vi "Host Main.vi"() -> ()   [LabVIEW 2014]
doc: "This application launches and executes the Tag Bus Data framework configuration for the specified target alias. This is a simple example of the framework API functions, but may also be a suitable starting point for a Host UI or Thick Client that is running a local version of the framework."
uses:
  <vilib>/NI/Module Execution Interface/Engine Runtime/Execution States.ctl
  <vilib>/NI/Module Execution Interface/Engine Runtime/Fault.ctl
  <vilib>/NI/Tag Bus Module Framework/runtime/error classification.ctl
  <vilib>/NI/Current Value Table/DataTypes/Double_Read.vi
  <vilib>/NI/Current Value Table/DataTypes/Array of Double_Read.vi
  <vilib>/NI/Current Value Table/Type to Enum.vi
  <vilib>/NI/Current Value Table/DataTypes/Double_Type To Enum.vi
  <vilib>/NI/Current Value Table/DataTypes/Array of Double_Type To Enum.vi
  <vilib>/NI/Current Value Table/FGVs/CVT Globals.vi
  <vilib>/NI/Current Value Table/FGVs/Tag Memory.vi
  <vilib>/NI/Current Value Table/Memory Block.vi
  <vilib>/NI/Current Value Table/DataTypes/Double_Memory Block.vi
  <vilib>/NI/Current Value Table/DataTypes/Array of Double_Memory Block.vi
  <vilib>/userdefined/High Color/nirio_resource_hc.ctl
  <vilib>/NI/Module Execution Interface/Engine Runtime/Engine Runtime Interface.lvclass
  <vilib>/NI/DCAF/Tag Editor Core/Framework Configuration Classes/target runtime/PL_Target Runtime.lvclass
  <vilib>/NI/Tag Bus Module Framework/FPGA manager/FPGA manager.lvlib
  <vilib>/rvi/interface/nirviOpenFPGA/nirviOpenFPGA.xnode
  <vilib>/NI/Tag Bus Module Framework/FPGA manager/methods.ctl
  <vilib>/NI/Current Value Table/Current Value Table.lvlib
  <vilib>/NI/Tag Bus Module Framework/runtime/TBM module execution interface.lvclass
panel:
  out "DiskUsage":dbl
  out "DiskUsagePercentage":dbl
  out "CPU_Usage":dbl[](array[numeric])
  out "CPU_UsageTotal":dbl
  out "MemoryUsagePercentage":dbl
  out "MemoryUsage":dbl
  out "engine status":T4(array[cluster])
  in  "stop":bool
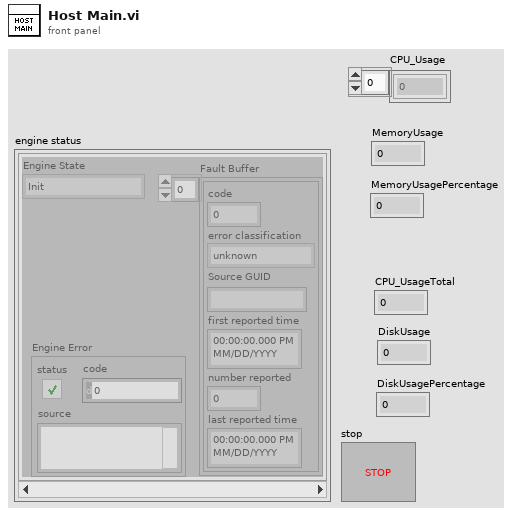
[diagram p1: front panel]
types:
  T1 = typedef "Engine Runtime Interface.lvclass/Execution States.ctl" = enum16{"Init", "Pre-Operational", "Safe-Operational", "Operational", "Stopped"}
  T2 = typedef "Engine Runtime Interface.lvclass/Fault.ctl" = cluster{"code":i32, "error classification":T3, "Source GUID":string, "first reported time":timestamp, "number reported":u32, "last reported time":timestamp}
  T3 = typedef "TBM module execution interface.lvclass/error classification.ctl" = enum16{"unknown", "none", "trivial", "recoverable", "critical"}
  T4 = cluster{"Engine State":T1, "Fault Buffer":T2[], "Engine Error":errorcluster}[]
  T5 = typedef "FPGA manager.lvlib/methods.ctl" = enum16{"initialize bitfile", "cache bitfile", "locate bitfile", "close bitfile", "clear manager"}
  T6 = typedef "nirio_resource_hc.ctl" = tag
  T7 = cluster{"Engine State":T1, "faults":T2[], "Engine Error":errorcluster}
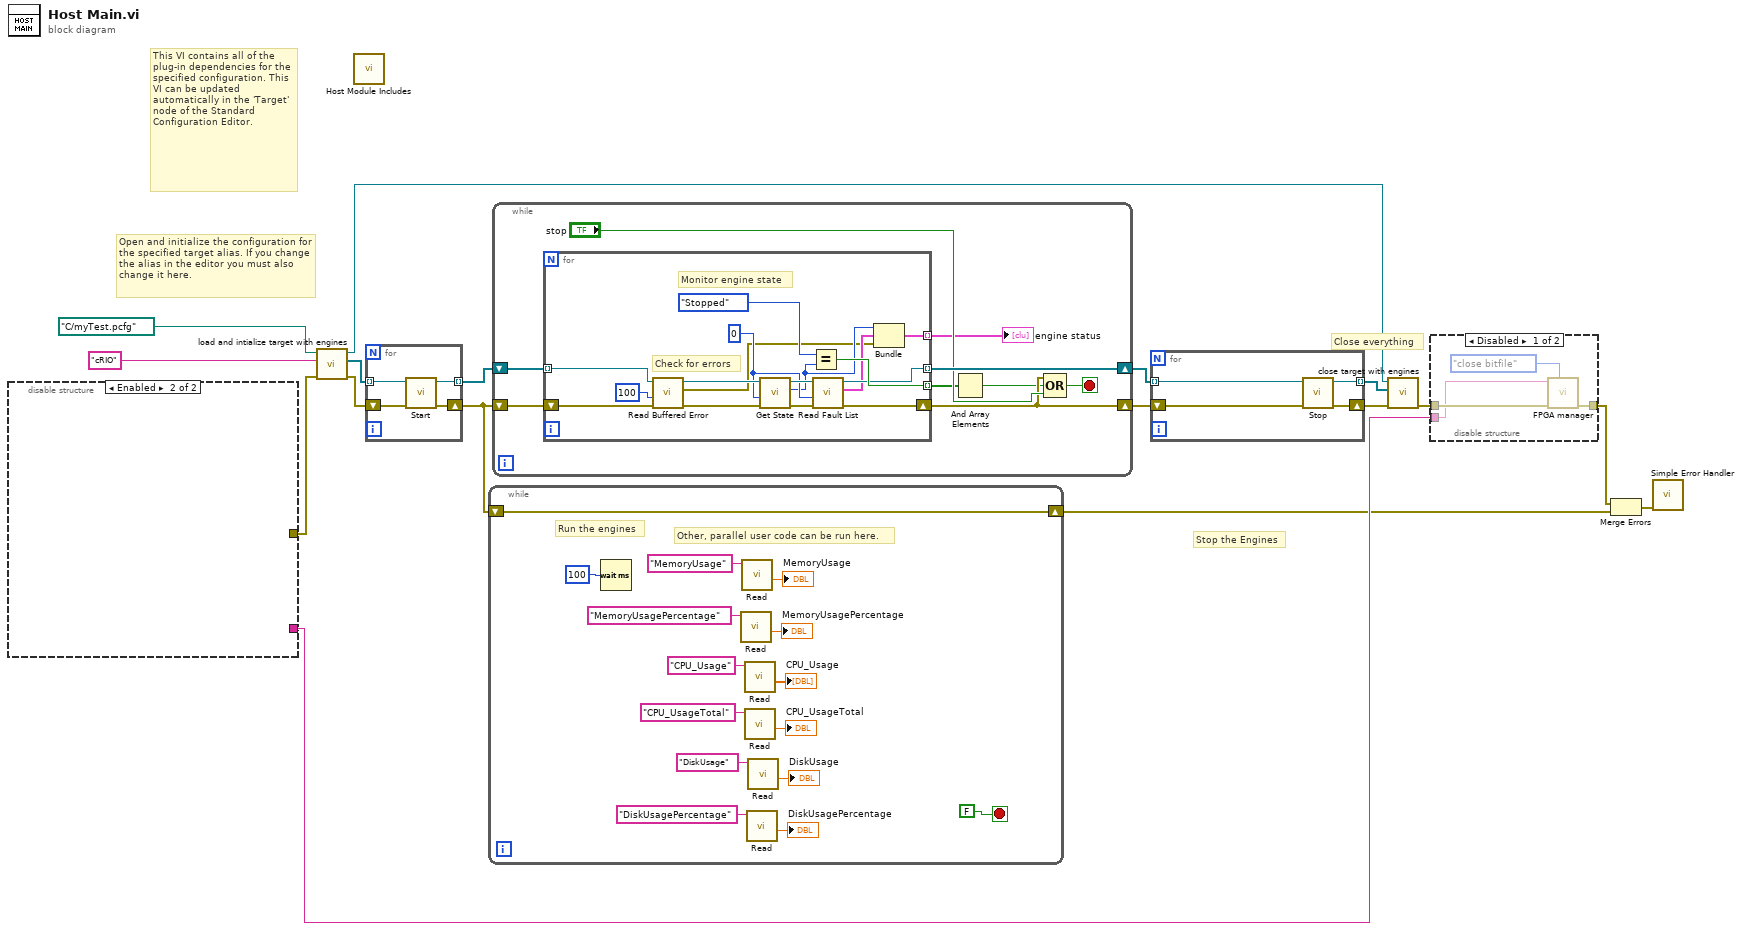
[diagram p0: block diagram]
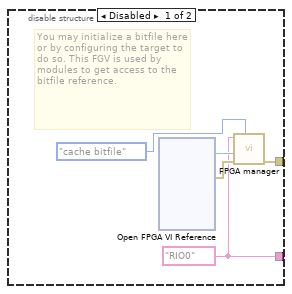
[diagram p3: hidden frame]
diagram:
  # "Open and initialize the configuration for the specified target alias. If you change the alias in the editor you must also change it here."
  # "Close everything"
  # "Stop the Engines"
  # "This VI contains all of the plug-in dependencies for the specified configuration. This VI can be updated automatically in the 'Target' node of the Standard Configuration Editor."
  # "Run the engines"
  n1 = disable-structure shown="Enabled" {
    disable-tunnel: [w22 _] -> w7
    disable-tunnel: [w18 _] -> w6
    frame Disabled {
      w18 = T6 "RIO0" ("RIO resource")
      # "You may initialize a bitfile here or by configuring the target to do so. This FGV is used by modules to get access to the bitfile reference."
      n2 = xnode "Open FPGA VI Reference"() -> ("FPGA VI Reference Out"=w20:refnum<k20>, "error out"=w21:errorcluster)  [unwired: 2 in]
      n3 = call <vilib>:"FPGA manager.vi"("action"=methods."cache bitfile", "error in"=w21, "bitfile to cache"=w20, "RIO resource"=w18) -> ("error out"=w22:errorcluster)  [unwired: 5 in, 2 out]
    }
    frame Enabled {
    }
  }
  n4 = call <vilib>:"load and intialize target with engines.vi"("error in"=w7, "target alias"="cRIO", "file path"=path "C:/myTest.pcfg" ("configuration file path")) -> ("error out"=w14:errorcluster, "engine runtime interfaces"=w13:refnum<class "Engine Runtime Interface.lvclass">[], "target runtime"=w10:refnum<class "PL_Target Runtime.lvclass">)  [unwired: 6 in]
  n5 = call "Host Module Includes.vi"() -> ()  [unwired: 12 in]
  n6 = for {
    tunnel: [w26] -> w17 mode=indexing
    tunnel: w13 -> [w23] mode=indexing
    shift-right: [w25] -> w5
    shift-left: w14 -> [w24]
    n7 = call-dynamic "Start.vi"("error in"=w24, "Engine Runtime Interface in"=w23) -> ("error out"=w25:errorcluster, "Engine Runtime Interface out"=w26:refnum<class "Engine Runtime Interface.lvclass">)  [unwired: 8 in]
  }
  n8 = while {
    shift-right: [w39] -> w4
    shift-left: w5 -> [w39]
    stop <- FALSE stop-if-true
    # "Other, parallel user code can be run here."
    n9 = Wait (ms)(milliseconds to wait=u32 100) -> ()  [unwired: 1 out]
    n10 = call-poly <vilib>:"Read.vi"("Tag Name"="MemoryUsagePercentage") -> ("Value"=→"MemoryUsagePercentage":dbl)  [unwired: 9 in, 1 out]
    n11 = call-poly <vilib>:"Read.vi"("Tag Name"="MemoryUsage") -> ("Value"=→"MemoryUsage":dbl)  [unwired: 9 in, 1 out]
    n12 = call-poly <vilib>:"Read.vi"("Tag Name"="CPU_Usage") -> ("Value"=→"CPU_Usage":dbl[])  [unwired: 9 in, 1 out]
    n13 = call-poly <vilib>:"Read.vi"("Tag Name"="CPU_UsageTotal") -> ("Value"=→"CPU_UsageTotal":dbl)  [unwired: 9 in, 1 out]
    n14 = call-poly <vilib>:"Read.vi"("Tag Name"="DiskUsagePercentage") -> ("Value"=→"DiskUsagePercentage":dbl)  [unwired: 9 in, 1 out]
    n15 = call-poly <vilib>:"Read.vi"("Tag Name"="DiskUsage") -> ("Value"=→"DiskUsage":dbl)  [unwired: 9 in, 1 out]
  }
  n16 = while {
    shift-right: [w48] -> w16
    shift-left: w17 -> [w50]
    shift-right: [w45] -> w15
    shift-left: w5 -> [w49]
    stop <- w46 stop-if-true
    n17 = for {
      tunnel: w50 -> [w66] mode=indexing
      tunnel: [w57] -> w48 mode=indexing
      tunnel: [w61] -> w43 mode=indexing
      shift-right: [w56] -> w45
      shift-left: w49 -> [w65]
      tunnel: [w51] -> w44 mode=indexing
      w55 = 0 ("timeout (-1)")
      # "Monitor engine state"
      # "Check for errors"
      n18 = call-dynamic "Read Buffered Error.vi"("error in"=w65, "timeout in ms (0)"=100, "Engine Runtime Interface in"=w66) -> ("error out"=w63:errorcluster, "Engine Error"=w52:errorcluster, "Engine Runtime Interface out"=w64:refnum<class "Engine Runtime Interface.lvclass">)  [unwired: 6 in]
      n19 = call-dynamic "Get State.vi"("error in"=w63, "timeout (-1)"=w55, "Engine Runtime Interface in"=w64) -> ("error out"=w59:errorcluster, "Engine State"=w54:T1, "Engine Runtime Interface out"=w58:refnum<class "Engine Runtime Interface.lvclass">)  [unwired: 6 in]
      n20 = Equal?(x=Execution_States."Stopped" ("Engine State"), y=w54) -> (x = y?=w61:bool)
      n21 = call-dynamic "Read Fault List.vi"("error in"=w59, "timeout (-1)"=w55, "Engine Runtime Interface in"=w58) -> ("error out"=w56:errorcluster, "faults"=w53:T2[], "Engine Runtime Interface out"=w57:refnum<class "Engine Runtime Interface.lvclass">)  [unwired: 6 in]
      n22 = Bundle("Engine State"=w54, "faults"=w53, "Engine Error"=w52) -> (w51:T7)  [unwired: 1 in]
    }
    "engine status" <- w44
    n23 = And Array Elements(Boolean array=w43) -> (logical AND=w42:bool)
    n24 = Compound Arithmetic op=OR(w45, w42, "stop") -> (w46:bool)
  }
  n25 = for {
    tunnel: w16 -> [w70] mode=indexing
    shift-right: [w67] -> w9
    shift-left: w15 -> [w69]
    tunnel: [w68] -> w11 mode=indexing
    n26 = call-dynamic "Stop.vi"("error in"=w69, "Engine Runtime Interface in"=w70) -> ("error out"=w67:errorcluster, "Engine Runtime Interface out"=w68:refnum<class "Engine Runtime Interface.lvclass">)  [unwired: 8 in]
  }
  n27 = call <vilib>:"close target with engines.vi"("error in"=w9, "Engine Runtime Interfaces"=w11, "Target Runtime"=w10) -> ("error out"=w3:errorcluster)  [unwired: 8 in]
  n28 = disable-structure shown="Disabled" {
    disable-tunnel: [w73 w75] -> w2
    disable-tunnel: w3 -> [w74 w75]
    disable-tunnel: w6 -> [w71 _]
    frame Disabled {
      n29 = call <vilib>:"FPGA manager.vi"("action"=methods."close bitfile", "error in"=w74, "RIO resource"=w71) -> ("error out"=w73:errorcluster)  [unwired: 6 in, 2 out]
    }
    frame Enabled {
    }
  }
  n30 = Merge Errors(w2, w4) -> (w1:errorcluster)
  n31 = call <vilib>:"Simple Error Handler.vi"("error in (no error)"=w1) -> ()  [unwired: 4 in, 5 out]
